vi "cache tag indices.vi"(8 "error in":errorcluster, 9 "index cluster":variant, 10 "channel classification":T1, 11 "fixed channel runtime in":refnum<class "Watchdog runtime.lvclass">) -> (0 "error out":errorcluster, 3 "fixed channel runtime out":refnum<class "Watchdog runtime.lvclass">)   [LabVIEW 2013, in "Watchdog runtime.lvclass"]
uses:
  Watchdog runtime.lvclass
  <vilib>/NI/Tag Bus Module Framework/channel/channel classification.ctl
  <vilib>/NI/Tag Bus Data Framework/control module/runtime/control module runtime.lvclass
  <vilib>/NI/Tag Bus Module Framework/channel/TBM channel.lvclass
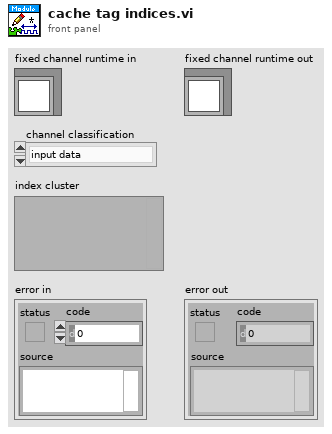
[diagram p1: front panel]
types:
  T1 = typedef "TBM channel.lvclass/channel classification.ctl" = enum16{"input data", "output data", "processing parameter", "processing result"}
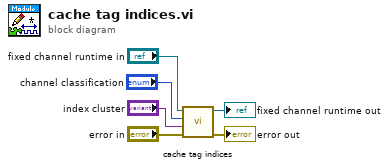
[diagram p0: block diagram]
diagram:
  n1 = call-parent "cache tag indices.vi"("error in"="error in", "index cluster"="index cluster", "channel classification"="channel classification", "fixed channel runtime in"="fixed channel runtime in") -> ("error out"=→"error out":errorcluster, "fixed channel runtime out"=→"fixed channel runtime out":refnum<class "Watchdog runtime.lvclass">)  [unwired: 6 in]
